vi "DrawHand.vi"(9 "Normalized Landmakers":u32[][](array[numeric]), 10 "New Image":T1, 11 "In Image":T1) -> (3 "Out Image":T1)   [LabVIEW 2024]
uses:
  <vilib>/vision/Image Controls.llb/IMAQ Image.ctl
panel:
  # "Landmarkers description"
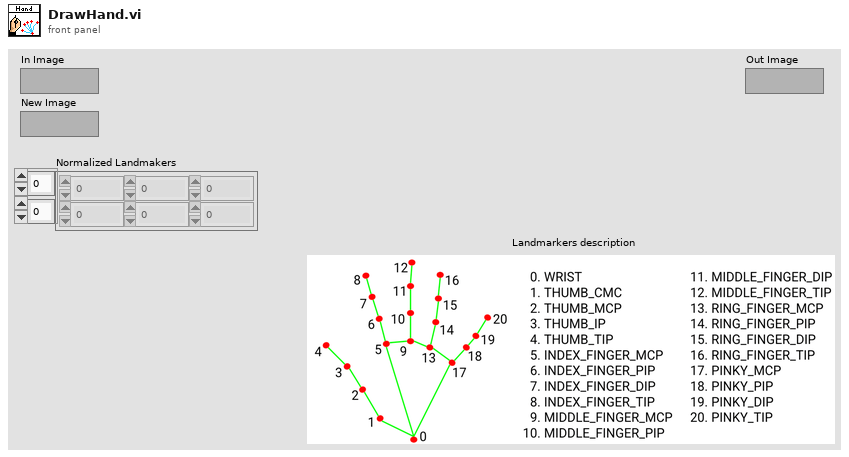
[diagram p1: front panel]
types:
  T1 = typedef "IMAQ Image.ctl" = refnum<image>
  T2 = cluster{"Red or Hue value":u8, "Green or Sat value":u8, "Blue or Luma or Val or Inten value":u8}
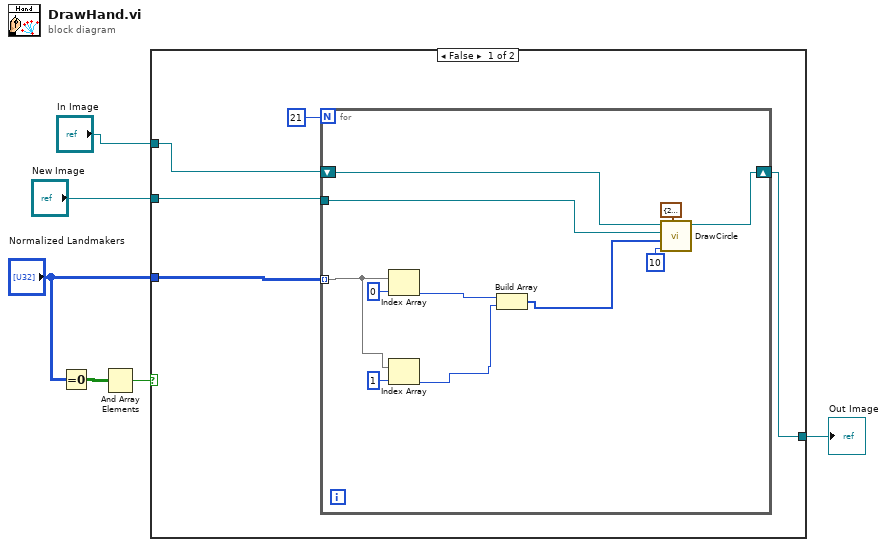
[diagram p0: block diagram]
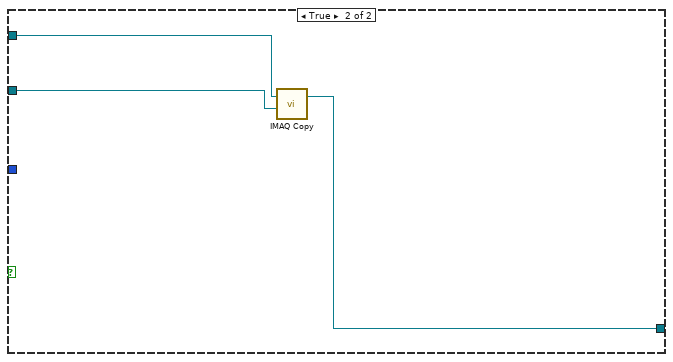
[diagram p2: hidden frame]
diagram:
  n1 = Equal To 0?(x="Normalized Landmakers") -> (x = 0?=w2:bool[][])
  n2 = And Array Elements(Boolean array=w2) -> (logical AND=w1:bool)
  n3 = case shown="False" w1 {
    tunnel: [w10 w23] -> w6
    tunnel: "New Image" -> [w9 w24]
    tunnel: "In Image" -> [w8 w25]
    tunnel: "Normalized Landmakers" -> [w7 _]
    frame False {
      n4 = for {
        N: 21 -> [_]
        tunnel: w7 -> [w20] mode=indexing
        tunnel: w9 -> [w16]
        shift-right: [w17] -> w10
        shift-left: w8 -> [w15]
        n5 = Index Array(array=w20, index=0) -> (element=w14:u32)
        n6 = Index Array(array=w20, index=1) -> (element=w13:u32)
        n7 = Build Array(w14, w13) -> (w12:u32[])
        n8 = call "DrawCircle.vi"("Color"=T2 {"Red or Hue value"=255, "Green or Sat value"=0, "Blue or Luma or Val or Inten value"=0}, "Radius"=u32 10, "Center coord"=w12, "New Image"=w16, "Refnum in"=w15) -> ("Refnum out"=w17:T1)  [unwired: 6 in]
      }
    }
    frame True {
      n9 = call "IMAQ Copy"("Image Dst"=w24, "Image Src"=w25) -> ("Image Dst Out"=w23:T1)  [unwired: 4 in, 1 out]
    }
  }
  "Out Image" <- w6
